vi "BuildComplexScanInputString.vi"(1 "Python String":string) -> (0 "Scan Input String":string)   [LabVIEW 2020, in "jki_python_data_tools.lvlib"]
uses:
  jki_python_data_tools.lvlib
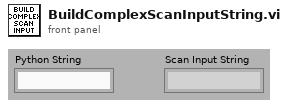
[diagram p1: front panel]
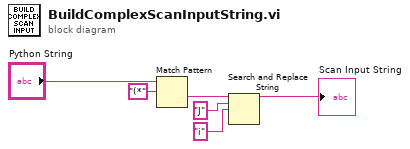
[diagram p0: block diagram]
diagram:
  n1 = Match Pattern(string="Python String", regular expression="(*") -> (after substring=w5:string)  [unwired: 1 in, 3 out]
  n2 = Search and Replace String(input string=w5, search string="J", replace string="i" ("replace string (\"\")")) -> (result string=→"Scan Input String":string)  [unwired: 5 in, 3 out]
